vi "swerve_raw_to_vec.vi"(8 "Raw Position BR":i32, 9 "Raw Position BL":i32, 10 "Raw Position FL":i32, 11 "Raw Position FR":i32) -> (2 "Output Matrix":T1)   [LabVIEW 2020]
uses:
  <vilib>/Analysis/Matrix/Datatypes/RealMatrix.ctl
  globals.vi
  <vilib>/Analysis/Matrix/NI_Matrix.lvlib
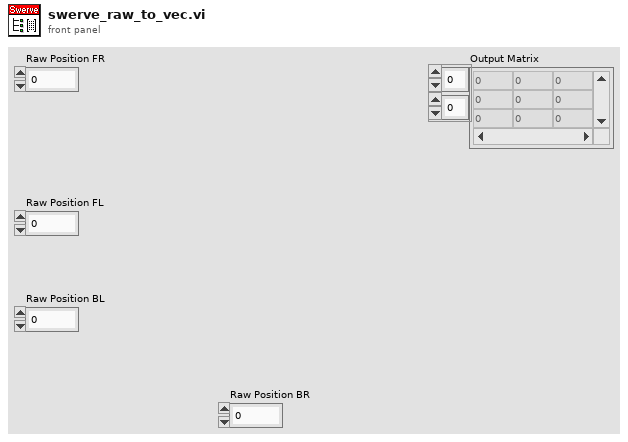
[diagram p1: front panel]
types:
  T1 = typedef "NI_Matrix.lvlib/RealMatrix.ctl" = dbl[][]
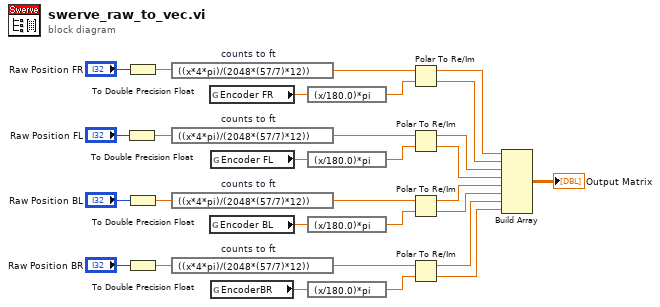
[diagram p0: block diagram]
diagram:
  n1 = To Double Precision Float(number="Raw Position FL") -> (double precision float=w2:dbl)
  n2 = To Double Precision Float(number="Raw Position FR") -> (double precision float=w1:dbl)
  n3 = To Double Precision Float(number="Raw Position BL") -> (double precision float=w4:dbl)
  n4 = To Double Precision Float(number="Raw Position BR") -> (double precision float=w3:dbl)
  n5 = expression code="((x*4*pi)/(2048*(57/7)*12))" "counts to ft"(w1) -> (w26:dbl)
  n6 = expression code="((x*4*pi)/(2048*(57/7)*12))" "counts to ft"(w2) -> (w27:dbl)
  n7 = expression code="((x*4*pi)/(2048*(57/7)*12))" "counts to ft"(w4) -> (w28:dbl)
  n8 = expression code="((x*4*pi)/(2048*(57/7)*12))" "counts to ft"(w3) -> (w29:dbl)
  n9 = global read "globals.vi" "Encoder FR"() -> (w16:dbl)
  n10 = global read "globals.vi" "Encoder BL"() -> (w14:dbl)
  n11 = global read "globals.vi" "Encoder FL"() -> (w15:dbl)
  n12 = global read "globals.vi" "EncoderBR"() -> (w13:dbl)
  n13 = expression code="(x/180.0)*pi" ("degrees to radians")(w16) -> (w9:dbl)
  n14 = expression code="(x/180.0)*pi" ("degrees to radians")(w15) -> (w10:dbl)
  n15 = expression code="(x/180.0)*pi" ("degrees to radians")(w14) -> (w11:dbl)
  n16 = expression code="(x/180.0)*pi" ("degrees to radians")(w13) -> (w12:dbl)
  n17 = Polar To Re/Im(2:w9, 3:w26) -> (0:w18:dbl, 1:w17:dbl)
  n18 = Polar To Re/Im(2:w10, 3:w27) -> (0:w20:dbl, 1:w19:dbl)
  n19 = Polar To Re/Im(2:w11, 3:w28) -> (0:w22:dbl, 1:w21:dbl)
  n20 = Polar To Re/Im(2:w12, 3:w29) -> (0:w24:dbl, 1:w23:dbl)
  n21 = Build Array(w17, w18, w19, w20, w21, w22, w23, w24) -> (→"Output Matrix":T1)
